vi "setUp.vi"(8 "error in (no error)":errorcluster, 11 "reference in":refnum<class "TestProtectedSubpanel.lvclass">) -> (0 "error out":errorcluster, 3 "reference out":refnum<class "TestProtectedSubpanel.lvclass">)   [LabVIEW 2017, in "TestProtectedSubpanel.lvclass"]
doc: "setUp runs prior to the test method during test execution. Use this method to initialize any object data required by your tests."
uses:
  TestProtectedSubpanel.lvclass
  <vilib>/addons/_JKI Toolkits/VI Tester/TestCase.llb/TestCase.lvclass
  <vilib>/ActorFramework/Actor/Actor.lvclass
  Doubles/ViewableDoubles/ViewableOne/ViewableOne.lvclass
  Doubles/ViewableDoubles/LeakyViewable/LeakyViewable.lvclass
  Doubles/ViewableDoubles/ViewableTwo/ViewableTwo.lvclass
  Doubles/ViewableDoubles/LeakyViewable/Leak Location.ctl
  C:/Git/mva-framework/Test/Doubles/ViewableDoubles/LeakyViewable/LeakyViewable.lvclass
  C:/Program Files (x86)/National Instruments/LabVIEW 2017/vi.lib/ActorFramework/Actor/Actor.lvclass
  C:/Program Files (x86)/National Instruments/LabVIEW 2017/vi.lib/addons/_JKI Toolkits/VI Tester/TestCase.llb/TestCase.lvclass
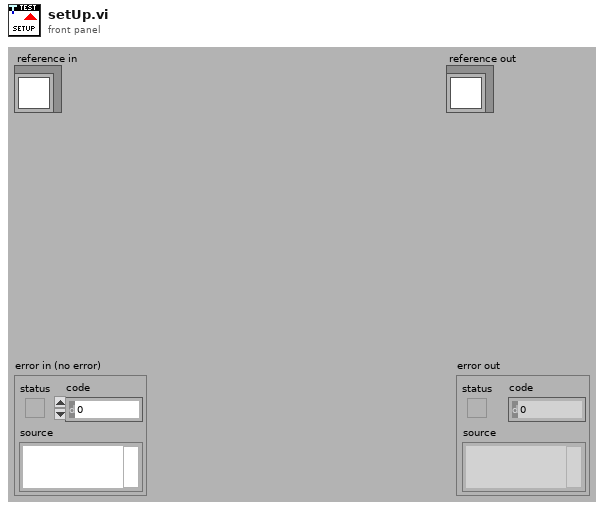
[diagram p1: front panel]
types:
  T1 = typedef "ViewableDoubles.lvlib/LeakyViewable.lvclass/Leak Location.ctl" = enum16{"Pre Launch Init", "Entering Actor Core", "Actor Core", "Exiting Actor Core", "Stop Core", "Handle Error"}
  T2 = cluster{"Location":T1, "State":refnum<class "IViewable.lvclass">, "Error Status":errorcluster}
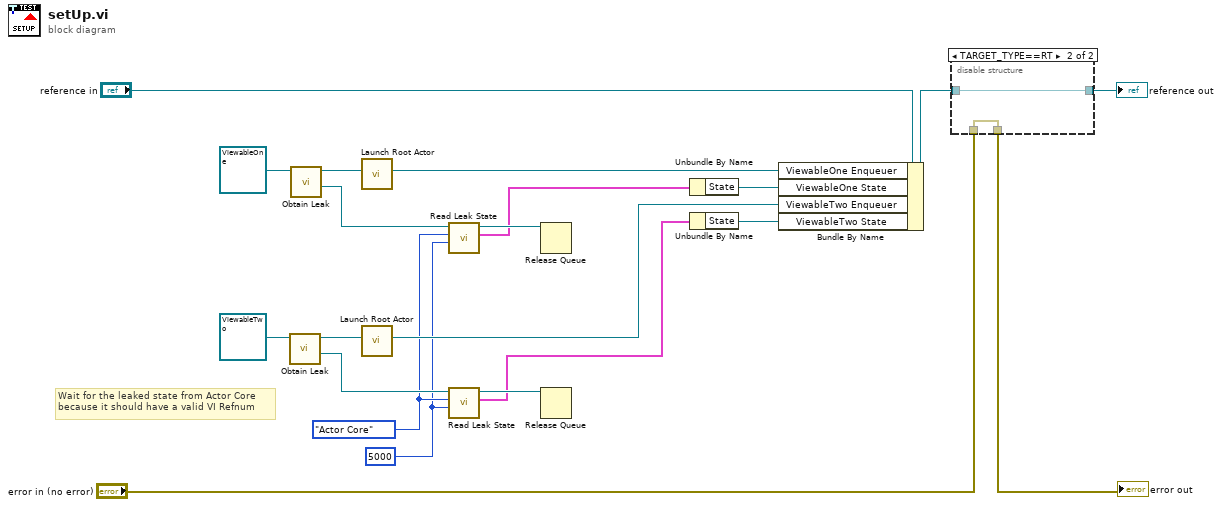
[diagram p0: block diagram]
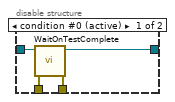
[diagram p2: hidden frame]
diagram:
  w2 = 5000 ("timeout in ms (-1)")
  w3 = Leak_Location."Actor Core" ("Leak Location")
  # "Wait for the leaked state from Actor Core\nbecause it should have a valid VI Refnum"
  n1 = call "Obtain Leak.vi"("LeakyViewable In"=refnum<class "ViewableTwo.lvclass"> refnum ("ViewableDoubles.lvlib:ViewableTwo.lvclass")) -> ("Viewable Leak Queue"=w4:refnum<queue>, "LeakyViewable Out"=w13:refnum<class "ViewableTwo.lvclass">)  [unwired: 9 in]
  n2 = call "Obtain Leak.vi"("LeakyViewable In"=refnum<class "ViewableOne.lvclass"> refnum ("ViewableDoubles.lvlib:ViewableOne.lvclass")) -> ("Viewable Leak Queue"=w8:refnum<queue>, "LeakyViewable Out"=w14:refnum<class "ViewableOne.lvclass">)  [unwired: 9 in]
  n3 = call <vilib>:"Launch Root Actor.vi"("Actor"=w14) -> ("Actor's Enqueuer"=w16:refnum<class "Message Enqueuer.lvclass">)  [unwired: 9 in, 1 out]
  n4 = call <vilib>:"Launch Root Actor.vi"("Actor"=w13) -> ("Actor's Enqueuer"=w15:refnum<class "Message Enqueuer.lvclass">)  [unwired: 9 in, 1 out]
  n5 = call "Read Leak State.vi"("timeout in ms (-1)"=w2, "Leak Location"=w3, "Viewable Leak Queue In"=w8) -> ("State Snapshot"=w6:T2, "Viewable Leak Queue"=w7:refnum<queue>)  [unwired: 5 in, 2 out]
  n6 = call "Read Leak State.vi"("timeout in ms (-1)"=w2, "Leak Location"=w3, "Viewable Leak Queue In"=w4) -> ("State Snapshot"=w1:T2, "Viewable Leak Queue"=w5:refnum<queue>)  [unwired: 5 in, 2 out]
  n7 = Release Queue(queue=w7) -> ()  [unwired: 2 in, 3 out]
  n8 = Release Queue(queue=w5) -> ()  [unwired: 2 in, 3 out]
  n9 = Unbundle By Name(w6) -> ("State"=w10:refnum<class "IViewable.lvclass">)
  n10 = Unbundle By Name(w1) -> ("State"=w9:refnum<class "IViewable.lvclass">)
  n11 = Bundle By Name(cluster="reference in", "ViewableOne Enqueuer"=w16, "ViewableOne State"=w10, "ViewableTwo Enqueuer"=w15, "ViewableTwo State"=w9) -> (w17:refnum<class "TestProtectedSubpanel.lvclass">)
  n12 = disable-structure shown="TARGET_TYPE==RT" {
    disable-tunnel: "error in (no error)" -> [w25 w26]
    disable-tunnel: [w24 w26] -> w20
    disable-tunnel: [w23 w27] -> w18
    disable-tunnel: w17 -> [w22 w27]
    frame condition #0 (active) {
      n13 = call <vilib>:"WaitOnTestComplete.vi"("error in (no error)"=w25, "TestCase in"=w22) -> ("error out"=w24:errorcluster, "TestCase out"=w23:refnum<class "TestProtectedSubpanel.lvclass">)  [unwired: 8 in]
    }
    frame condition #1 {
    }
  }
  "error out" <- w20
  "reference out" <- w18
